vi "SetParam.vi"(8 "error in (no error)":errorcluster caption="entrée d'erreur (pas d'erreur)", 10 "fetch_olivetti_faces":T1={"shuffle"=FALSE, "random_state"=0, "download_if_missing"=TRUE, "Returns"="Data"} {"random_state" min=-1}, 11 "Olivetti_faces.lvclass":refnum<class "Olivetti_faces.lvclass">) -> (0 "error out":errorcluster caption="sortie d'erreur", 3 "Olivetti_faces.lvclass":refnum<class "Olivetti_faces.lvclass">)   [LabVIEW 2020, in "Olivetti_faces.lvclass"]
doc: "Set Parameters"
uses:
  Olivetti_faces.lvclass
  Olivetti_faces.lvclass/Olivetti_faces.ctl
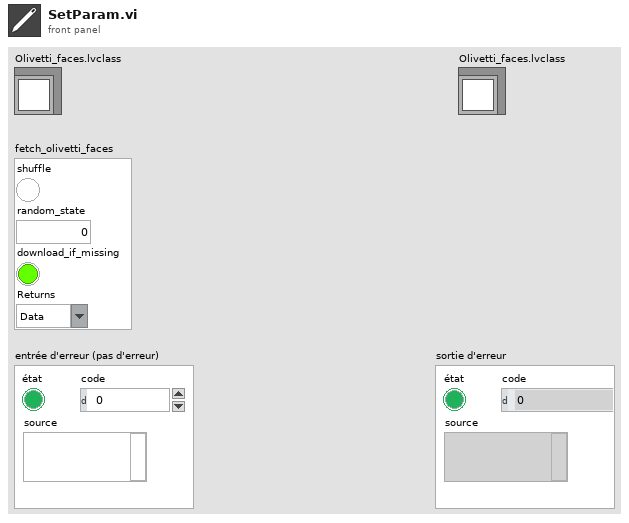
[diagram p1: front panel]
types:
  T1 = cluster{"shuffle":bool, "random_state":i32, "download_if_missing":bool, "Returns":string}
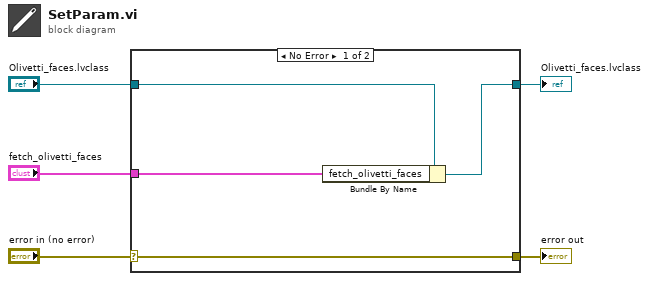
[diagram p0: block diagram]
diagram:
  n1 = case shown="No Error" "error in (no error)" {
    selector: "error in (no error)" -> [w9 w10]
    tunnel: [w9 w10] -> w4
    tunnel: [w7 w11] -> w2
    tunnel: "Olivetti_faces.lvclass" -> [w8 w11]
    tunnel: "fetch_olivetti_faces" -> [w6 _]
    frame No Error {
      n2 = Bundle By Name(cluster=w8, "fetch_olivetti_faces"=w6) -> (w7:refnum<class "Olivetti_faces.lvclass">)
    }
    frame Error {
    }
  }
  "error out" <- w4
  "Olivetti_faces.lvclass" <- w2
